vi "pw.vi"(5 "username":string, 9 "password":string, 11 "error in (no error)":errorcluster) -> (6 "ValidateCredentials":bool, 15 "error out":errorcluster)   [LabVIEW 2016]
uses:
  System.DirectoryServices.AccountManagement
panel:
  in  "options":T1(ring)=enum."SimpleBind"
  in  "name":string
  in  "contextType":i32(ring)=1 items=["Machine", "Domain", "ApplicationDirectory"]
  # "Settings specific to your windows domain setup"
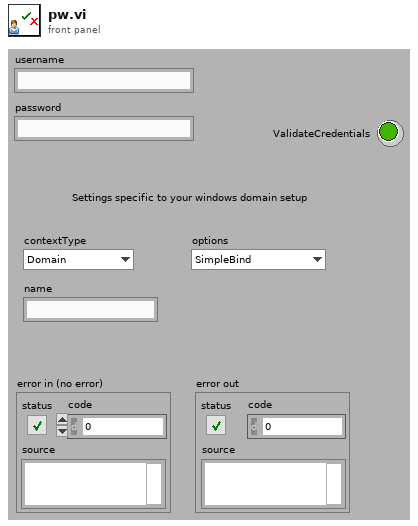
[diagram p1: front panel]
types:
  T1 = enum16{"Negotiate", "SimpleBind", "SecureSocketLayer", "Signing", "Sealing", "ServerBind"}
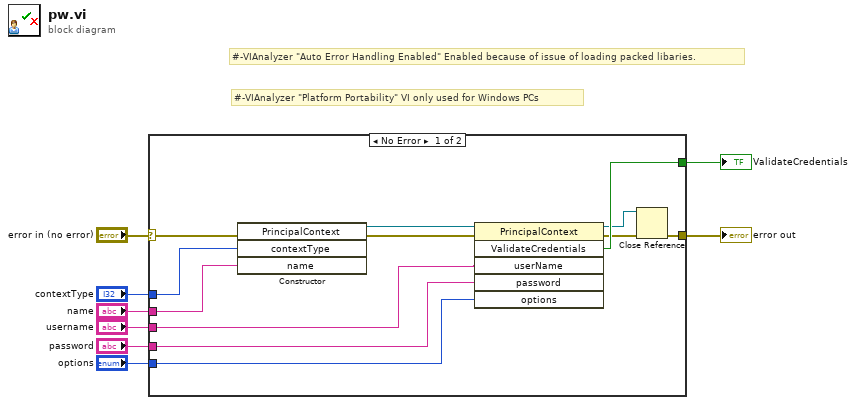
[diagram p0: block diagram]
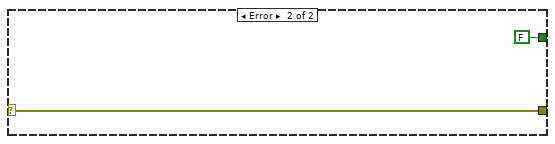
[diagram p2: hidden frame]
diagram:
  # "#-VIAnalyzer \"Platform Portability\" VI only used for Windows PCs"
  # "#-VIAnalyzer \"Auto Error Handling Enabled\" Enabled because of issue of loading packed libaries."
  n1 = case shown="No Error" "error in (no error)" {
    selector: "error in (no error)" -> [w9 w22]
    tunnel: "contextType" -> [w20 _]
    tunnel: "name" -> [w19 _]
    tunnel: "password" -> [w17 _]
    tunnel: [w16 FALSE ("ValidateCredentials")] -> w5
    tunnel: "options" -> [w15 _]
    tunnel: [w14 w22] -> w3
    tunnel: "username" -> [w12 _]
    frame No Error {
      n2 = constructor class="PrincipalContext"(error in=w9, "contextType"=w20, "name"=w19) -> (reference out=w18:refnum<k24>, error out=w13:errorcluster)  [unwired: 2 in, 3 out]
      n3 = invoke class="PrincipalContext" method="ValidateCredentials"(reference=w18, error in=w13, "userName"=w12, "password"=w17, "options"=w15) -> (reference out=w11:refnum<k24>, error out=w10:errorcluster, "ValidateCredentials"=w16:bool)  [unwired: 1 in, 3 out]
      n4 = Close Reference(reference=w11, error in (no error)=w10) -> (error out=w14:errorcluster)
    }
    frame Error {
    }
  }
  "ValidateCredentials" <- w5
  "error out" <- w3
